vi "Set Callback On Server Stopped.vi"(10 "OnServerStopped":cluster{}, 11 "index":u16) -> (3 "function return":i32)   [LabVIEW 2025, in "ExtremelyEpicImagerIPC2.lvlib"]
doc: "IMAGERIPC_API HRESULT WINAPI SetCallback_OnServerStopped(WORD index, fpOnServerStopped OnServerStopped);"
uses:
  ExtremelyEpicImagerIPC2.lvlib
  ImagerIPC2.dll
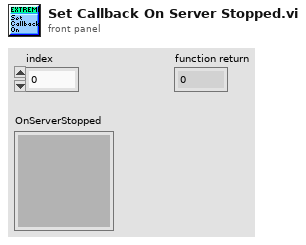
[diagram p1: front panel]
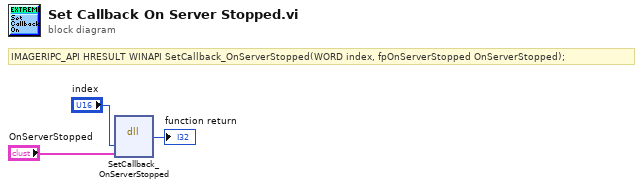
[diagram p0: block diagram]
diagram:
  # "IMAGERIPC_API HRESULT WINAPI SetCallback_OnServerStopped(WORD index, fpOnServerStopped OnServerStopped);"
  n1 = dll-call lib="C:/Users/mayhe/OneDrive/Documents/GitHub/In-situ-monitoring-of-powder-bed-fusion-additive-manufacturing/system_development/Orichalcum/v0.2/Software_design/thermal-camera/VI/Connect SDK/ImagerIPC2.*" fn="SetCallback_OnServerStopped"("index"="index", "OnServerStopped"="OnServerStopped") -> (→"function return":i32)  [unwired: 5 in, 2 out]
